vi "test-DiffDriveSim-current.vi"() -> (3 "Test Passed":bool)   [LabVIEW 2019]
uses:
  <vilib>/Rock Robotics/WPI/ThirdParty/JAS_Junk/TrajLib/DCMOTOR.CTL
  <vilib>/Rock Robotics/WPI/ThirdParty/JAS_Junk/TrajLib/LINEAR_SYSTEM.ctl
  <vilib>/Analysis/Matrix/Datatypes/RealMatrix.ctl
  <vilib>/Rock Robotics/WPI/ThirdParty/JAS_Junk/TrajLib/DIFF_DRIVE_TRAIN_SIM.ctl
  <vilib>/Rock Robotics/WPI/ThirdParty/JAS_Junk/TrajLib/DIFF_DRIVE_ToughBoxMini_MotorChoice_ENUM.ctl
  <vilib>/Rock Robotics/WPI/ThirdParty/JAS_Junk/TrajLib/MatBuilder_Create.vi
  <vilib>/Rock Robotics/WPI/ThirdParty/JAS_Junk/TrajLib/LinearSystem_New.vi
  <vilib>/Rock Robotics/WPI/ThirdParty/JAS_Junk/TrajLib/MatBuilder_Fill.vi
  <vilib>/Rock Robotics/WPI/ThirdParty/JAS_Junk/TrajLib/MatrixHelper_Zero.vi
  <vilib>/Rock Robotics/WPI/ThirdParty/JAS_Junk/TrajLib/MatrixHelper_CoerceSize.vi
  <vilib>/Rock Robotics/WPI/ThirdParty/JAS_Junk/TrajLib/Trajectory_Library.lvlib
  <vilib>/Analysis/Matrix/NI_Matrix.lvlib
panel:
  in  "Tab Control":T1(tab)
  out "Left Motor Vel (PV)":dbl format="%20.3f"
  out "Right Motor Vel (PV)":dbl format="%20.3f"
  out "CO Chart":cluster{"Voltage":dbl}(graph)
  out "PV Chart":T2(graph)
  out "Motor Amps":dbl format="%20.3f"
  out "Sim Upd Err":bool
  out "Lin Sys Size Cooerced":bool
  out "Cur Passed 0":bool
  out "Cur Passed 1":bool
  out "Cur Passed 2":bool
  out "DiffDriveMotor":T3 {"Jr_KgM2" format="%13.5p"; "L_H" format="%13.5p"; "Kt_NMPerAmp" format="%13.5p"; "KvINV_RadPerSecPerVolt" format="%13.5p"; "R_Ohms" format="%13.5p"; "FreeSpeed_RadPerSec" format="%13.5p"; "FreeCurrent_Amps" format="%13.5p"; "StallCurrent_Amps" format="%13.5p"; "StallTorque_NM" format="%13.5p"; "nominalVoltage_Volts" format="%13.5p"}
  out "m_DiffDriveVel":T4
  out "Differential Drive Train Sim":T6 {"m_Motor"."Jr_KgM2" format="%13.5p"; "m_Motor"."L_H" format="%13.5p"; "m_Motor"."Kt_NMPerAmp" format="%13.5p"; "m_Motor"."KvINV_RadPerSecPerVolt" format="%13.5p"; "m_Motor"."R_Ohms" format="%13.5p"; "m_Motor"."FreeSpeed_RadPerSec" format="%13.5p"; "m_Motor"."FreeCurrent_Amps" format="%13.5p"; "m_Motor"."StallCurrent_Amps" format="%13.5p"; "m_Motor"."StallTorque_NM" format="%13.5p"; "m_Motor"."nominalVoltage_Volts" format="%13.5p"}
  # "<States,States>"
  # "<States,Inputs>"
  # "<Outputs,States>"
  # "<Outputs,Inputs>"
  # "<States, 1>"
  # "<Outputs, 1>"
  # "<Inputs, 1>"
  # "<Outputs, 1>"
  # "<States,States>"
  # "<States,Inputs>"
  # "<Outputs,States>"
  # "<Outputs,Inputs>"
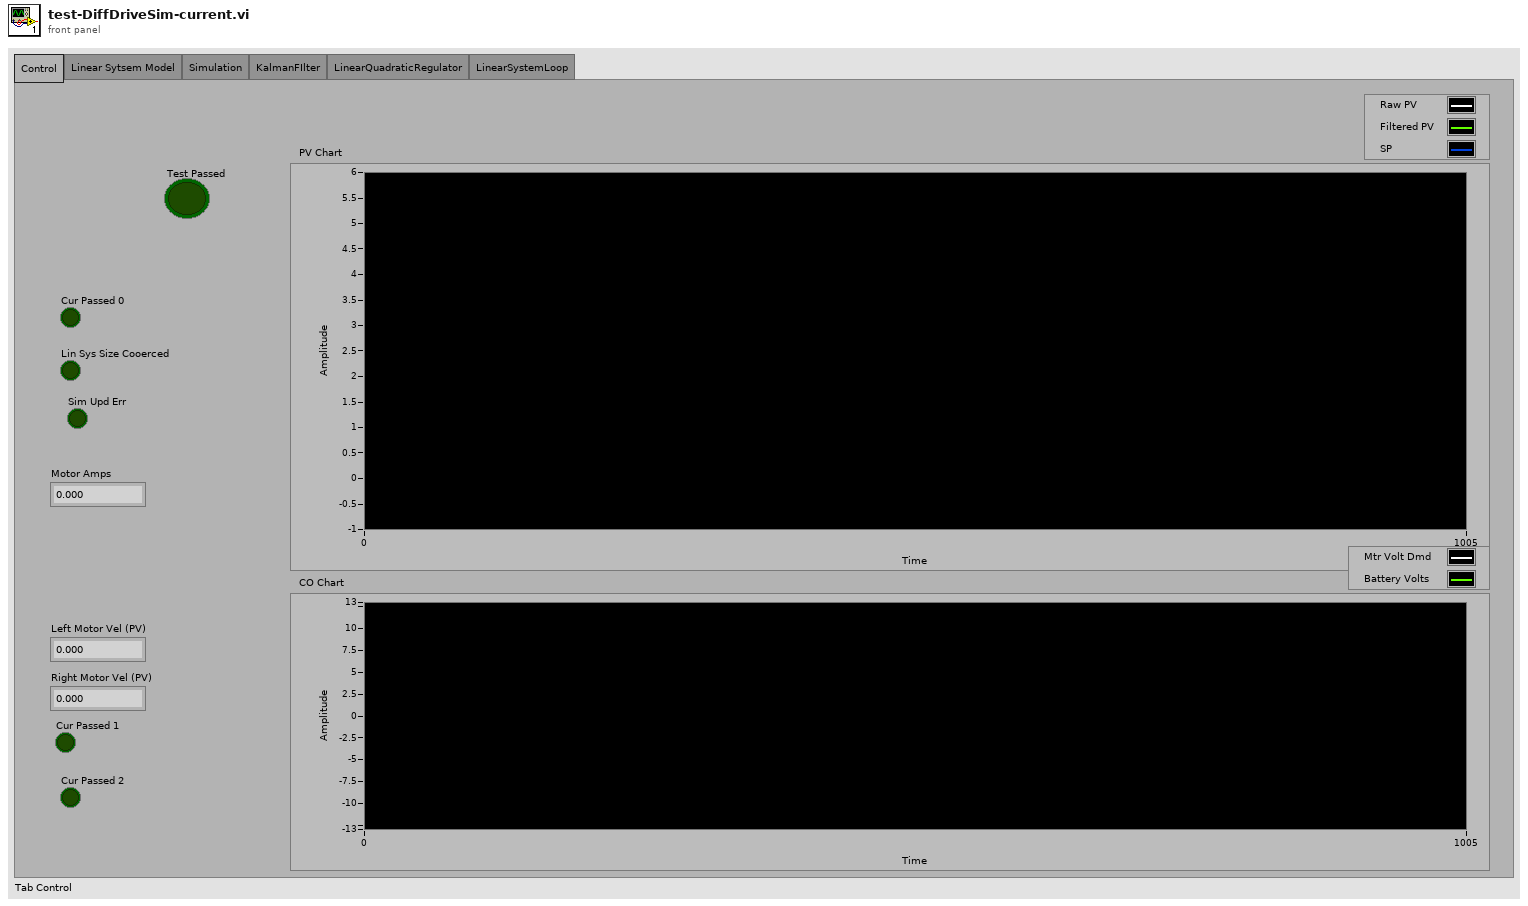
[diagram p1: front panel]
types:
  T1 = enum32{"Control", "Linear Sytsem Model", "Simulation", "KalmanFIlter", "LinearQuadraticRegulator", "LinearSystemLoop"}
  T2 = cluster{"LeftVelocity_M_Per_Sec":dbl, "RightVel_M_Per_Sec":dbl}
  T3 = typedef "Trajectory_Library.lvlib/DCMOTOR.CTL" = cluster{"nominalVoltage_Volts":dbl, "StallTorque_NM":dbl, "StallCurrent_Amps":dbl, "FreeCurrent_Amps":dbl, "FreeSpeed_RadPerSec":dbl, "R_Ohms":dbl, "KvINV_RadPerSecPerVolt":dbl, "Kt_NMPerAmp":dbl, "L_H":dbl, "Jr_KgM2":dbl}
  T4 = typedef "Trajectory_Library.lvlib/LINEAR_SYSTEM.ctl" = cluster{"m_A":T5, "m_B":T5, "m_C":T5, "m_D":T5, "States":i32, "Inputs":i32, "Outputs":i32}
  T5 = typedef "NI_Matrix.lvlib/RealMatrix.ctl" = dbl[][]
  T6 = typedef "Trajectory_Library.lvlib/DIFF_DRIVE_TRAIN_SIM.ctl" = cluster{"m_Plant":T4, "m_X":T5, "m_Y":T5, "m_U":T5, "MeasureStdDev":T5, "m_Motor":T3, "m_OriginalGearing":dbl, "m_CurrentGearing":dbl, "m_WheelRadius_M":dbl, "m_RB":dbl}
  T7 = typedef "Trajectory_Library.lvlib/DIFF_DRIVE_ToughBoxMini_MotorChoice_ENUM.ctl" = enum16{"One CIM Per Side", "Two CIM Per Side", "One MiniCIM Per Side", "Two Mini CIM Per Side", "Two Falcon Per Side", "Two NEO Per Side"}
  T8 = typedef "Trajectory_Library.lvlib/POSE2D.ctl" = cluster{"TRANSLATION":T9, "ROTATION":T10}
  T9 = typedef "Trajectory_Library.lvlib/TRANSLATION2D.ctl" = cluster{"X":dbl, "Y":dbl}
  T10 = typedef "Trajectory_Library.lvlib/ROTATION2D.ctl" = cluster{"VALUE":dbl, "COS":dbl, "SIN":dbl}
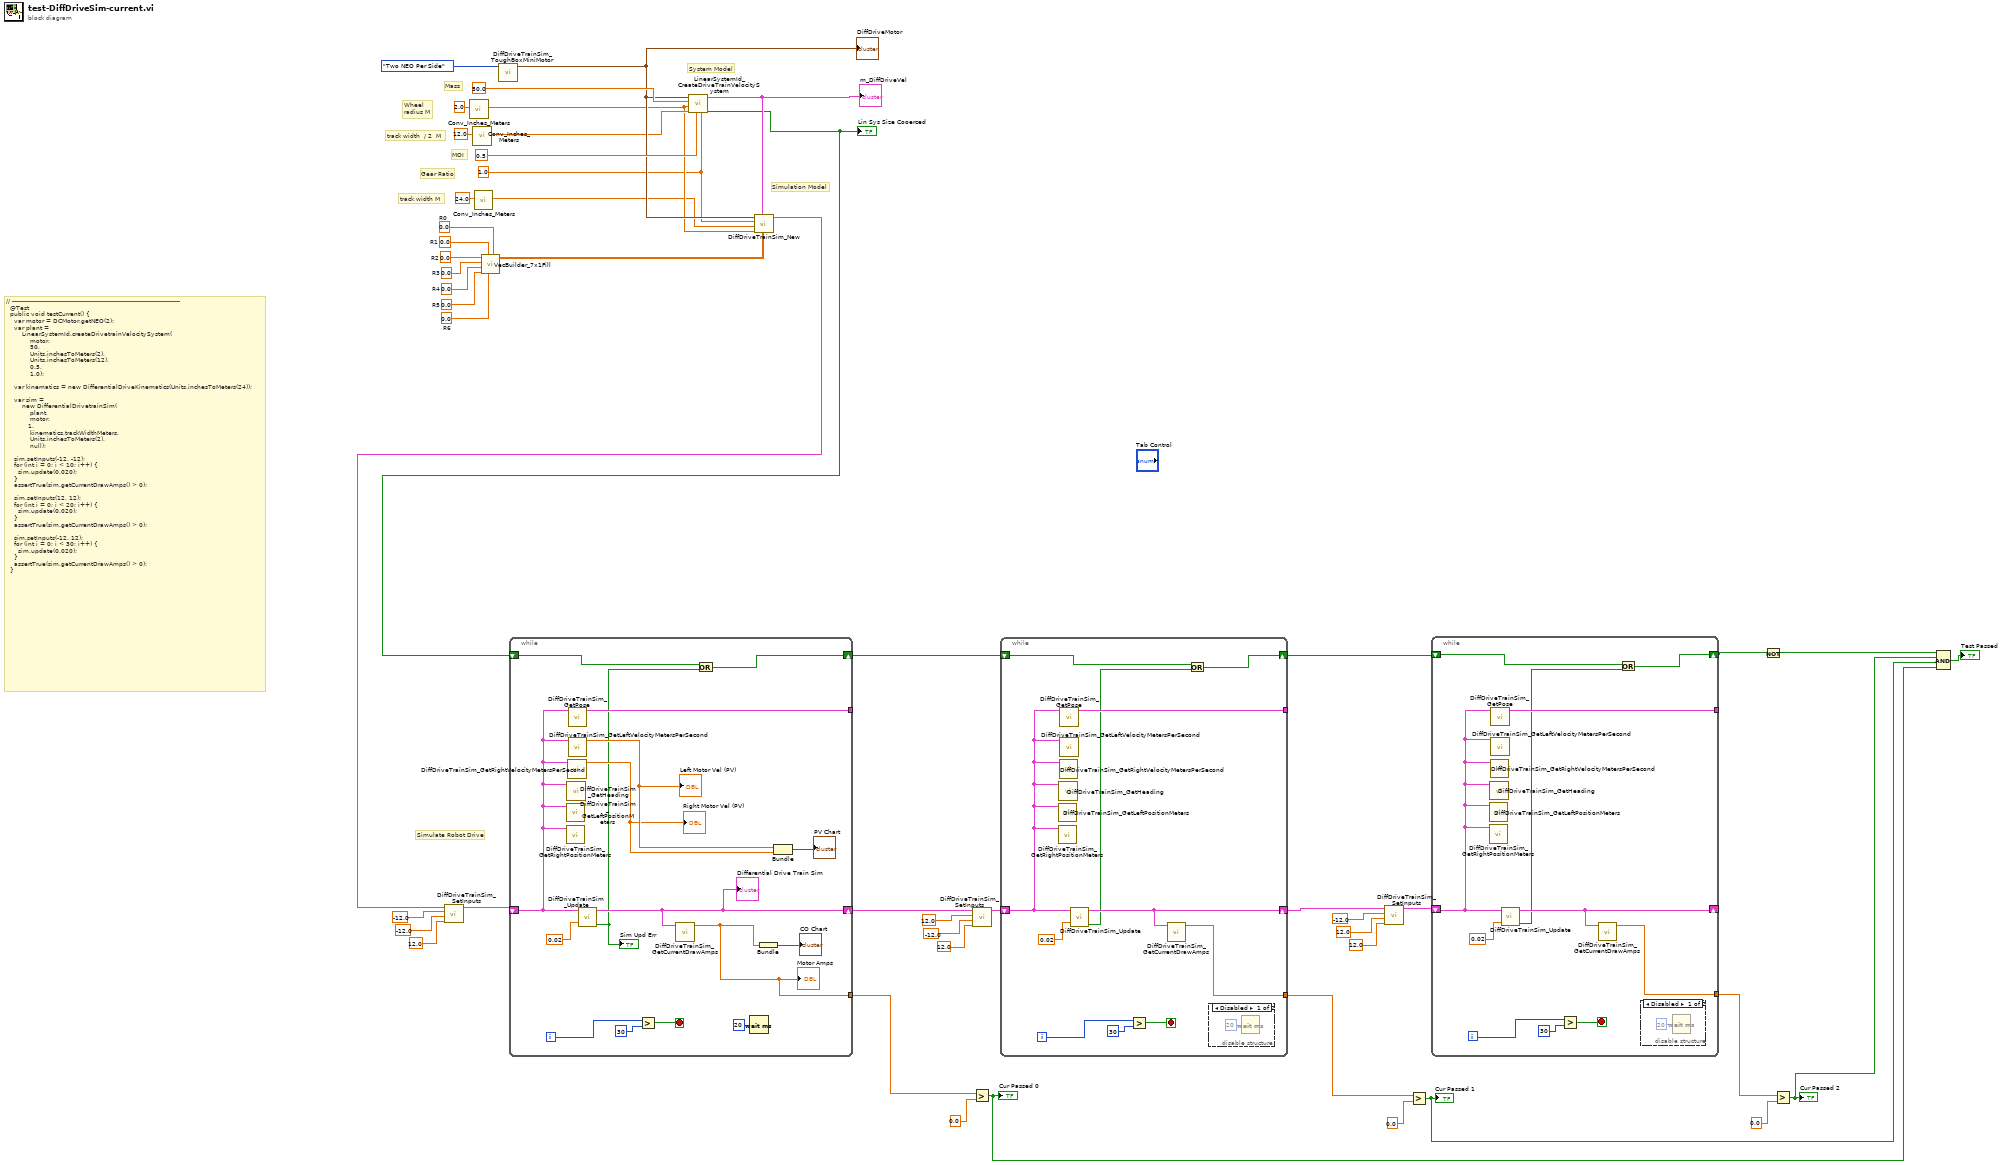
[diagram p0: block diagram]
diagram:
  w38 = 0.0  # R6
  w37 = 0.0  # R5
  w36 = 0.0  # R4
  w35 = 0.0  # R3
  w34 = 0.0  # R2
  w33 = 0.0  # R1
  w32 = 0.0  # R0
  w41 = 1.0 ("G")
  # "// ------------------------------------------------------------------------------------\n  @Test\n  public void testCurrent() {\n    var motor = DCMotor.getNEO(2);\n    var plant =\n        LinearSystemId.createDrivetrainVelocitySystem(\n            motor, \n            50, \n            Units.inchesToMeters(2), \n            Units.inchesToMeters(12), \n            0.5, \n            1.0);\n\n    var kinematics = new DifferentialDriveKinematics(Units.inchesToMeters(24));\n\n    var sim =\n        new DifferentialDrivetrainSim(\n            plant, \n            motor, \n           1, \n            kinematics.trackWidthMeters, \n            Units.inchesToMeters(2), \n            null);\n\n    sim.setInputs(-12, -12);\n    for (int i = 0; i < 10; i++) {\n      sim.update(0.020);\n    }\n    assertTrue(sim.getCurrentDrawAmps() > 0);\n\n    sim.setInputs(12, 12);\n    for (int i = 0; i < 20; i++) {\n      sim.update(0.020);\n    }\n    assertTrue(sim.getCurrentDrawAmps() > 0);\n\n    sim.setInputs(-12, 12);\n    for (int i = 0; i < 30; i++) {\n      sim.update(0.020);\n    }\n    assertTrue(sim.getCurrentDrawAmps() > 0);\n  }"
  # "track width M"
  # "Gear Ratio"
  # "Wheel\nradius M"
  # "track width  / 2  M"
  # "MOI"
  # "Simulation Model"
  # "System Model"
  # "Mass"
  # "Simulate Robot Drive"
  n1 = call <vilib>:"Conv_Inches_Meters.vi"("INCH"=2.0) -> ("Meters"=w43:dbl)  [unwired: 10 in]
  n2 = call <vilib>:"Conv_Inches_Meters.vi"("INCH"=12.0) -> ("Meters"=w44:dbl)  [unwired: 10 in]
  n3 = call <vilib>:"Conv_Inches_Meters.vi"("INCH"=24.0) -> ("Meters"=w39:dbl)  [unwired: 10 in]
  n4 = call <vilib>:"VecBuilder_7x1Fill.vi"("R0"=w32, "R6"=w38, "R1"=w33, "R5"=w37, "R4"=w36, "R3"=w35, "R2"=w34) -> ("output matrix"=w31:T5)  [unwired: 4 in]
  n5 = call <vilib>:"DiffDriveTrainSim_ToughBoxMiniMotor.vi"("ToughBoxMiniMotor"=DIFF_DRIVE_ToughBoxMini_MotorChoice_ENUM."Two NEO Per Side") -> ("DriveMotor"=w45:T3)  [unwired: 10 in]
  "DiffDriveMotor" <- w45
  n6 = call <vilib>:"LinearSystemId_CreateDriveTrainVelocitySystem.vi"("G"=w41, "JKgMetersSquared"=0.5 ("Mass_Kg"), "rbMeters"=w44, "rMeters"=w43, "MassKg"=50.0 ("Mass_Kg"), "Motor"=w45) -> ("Size Coerced"=w24:bool, "Linearsystem"=w42:T4)  [unwired: 4 in]
  "m_DiffDriveVel" <- w42
  "Lin Sys Size Cooerced" <- w24
  n7 = call <vilib>:"DiffDriveTrainSim_New.vi"("MeasurementStdDev"=w31, "DriveTrainPlant"=w42, "WheelRadius_M"=w43, "TrackWidth_M"=w39, "Gearing"=w41, "DriveMotor"=w45) -> ("DiffDriveTrainSim"=w30:T6)  [unwired: 5 in]
  n8 = call <vilib>:"DiffDriveTrainSim_SetInputs.vi"("BatteryVoltage"=12.0, "Right_Volts"=-12.0, "Left_Volts"=-12.0, "in DiffDriveTrainSim"=w30) -> ("out DiffDriveTrainSim"=w29:T6)  [unwired: 6 in, 1 out]
  n9 = while {
    shift-right: [w64] -> w14
    shift-left: w29 -> [w62]
    tunnel: [w55] -> _
    shift-right: [w52] -> w6
    shift-left: w24 -> [w53]
    tunnel: [w51] -> w21
    i -> [w60]
    stop <- w58 stop-if-true
    n10 = call <vilib>:"DiffDriveTrainSim_GetLeftPositionMeters.vi"("DiffDriveTrainSim"=w62) -> ()  [unwired: 10 in, 1 out]
    n11 = call <vilib>:"DiffDriveTrainSim_GetRightPositionMeters.vi"("DiffDriveTrainSim"=w62) -> ()  [unwired: 10 in, 1 out]
    n12 = call <vilib>:"DiffDriveTrainSim_GetHeading.vi"("DiffDriveTrainSim"=w62) -> ()  [unwired: 10 in, 1 out]
    n13 = call <vilib>:"DiffDriveTrainSim_GetRightVelocityMetersPerSecond.vi"("DiffDriveTrainSim"=w62) -> ("RightVel_M_Per_Sec"=w57:dbl)  [unwired: 10 in]
    "Right Motor Vel (PV)" <- w57
    n14 = call <vilib>:"DiffDriveTrainSim_GetPose.vi"("DiffDriveTrainSim"=w62) -> ("Pose"=w55:T8)  [unwired: 10 in]
    n15 = call <vilib>:"DiffDriveTrainSim_GetLeftVelocityMetersPerSecond.vi"("DiffDriveTrainSim"=w62) -> ("LeftVelocity_M_Per_Sec"=w63:dbl)  [unwired: 10 in]
    "Left Motor Vel (PV)" <- w63
    n16 = call <vilib>:"DiffDriveTrainSim_Update.vi"("dT_Seconds"=0.02, "in DiffDriveTrainSim"=w62) -> ("Error"=w54:bool, "out DiffDriveTrainSim"=w64:T6)  [unwired: 8 in]
    "Sim Upd Err" <- w54
    "Differential Drive Train Sim" <- w64
    n17 = Greater?(x=w60, y=30) -> (0:w58:bool)
    n18 = call <vilib>:"DiffDriveTrainSim_GetCurrentDrawAmps.vi"("DiffDriveTrainSim"=w64) -> ("TotalCurrent_Amps"=w51:dbl)  [unwired: 10 in]
    "Motor Amps" <- w51
    n19 = Or(x=w53, y=w54) -> (x .or. y?=w52:bool)
    n20 = Wait (ms)(milliseconds to wait=u32 20) -> ()  [unwired: 1 out]
    n21 = Bundle("TotalCurrent_Amps"=w51) -> (→"CO Chart":cluster{"TotalCurrent_Amps":dbl})  [unwired: 1 in]
    n22 = Bundle("LeftVelocity_M_Per_Sec"=w63, "RightVel_M_Per_Sec"=w57) -> (→"PV Chart":T2)  [unwired: 1 in]
  }
  n23 = call <vilib>:"DiffDriveTrainSim_SetInputs.vi"("BatteryVoltage"=12.0, "Right_Volts"=-12.0, "Left_Volts"=12.0, "in DiffDriveTrainSim"=w14) -> ("out DiffDriveTrainSim"=w13:T6)  [unwired: 6 in, 1 out]
  n24 = Greater?(x=w21, y=0.0) -> (0:w1:bool)
  "Cur Passed 0" <- w1
  n25 = while {
    shift-right: [w76] -> w12
    shift-left: w13 -> [w75]
    tunnel: [w71] -> _
    shift-right: [w68] -> w5
    shift-left: w6 -> [w69]
    tunnel: [w67] -> w8
    i -> [w74]
    stop <- w72 stop-if-true
    n26 = call <vilib>:"DiffDriveTrainSim_GetLeftPositionMeters.vi"("DiffDriveTrainSim"=w75) -> ()  [unwired: 10 in, 1 out]
    n27 = call <vilib>:"DiffDriveTrainSim_GetRightPositionMeters.vi"("DiffDriveTrainSim"=w75) -> ()  [unwired: 10 in, 1 out]
    n28 = call <vilib>:"DiffDriveTrainSim_GetHeading.vi"("DiffDriveTrainSim"=w75) -> ()  [unwired: 10 in, 1 out]
    n29 = call <vilib>:"DiffDriveTrainSim_GetRightVelocityMetersPerSecond.vi"("DiffDriveTrainSim"=w75) -> ()  [unwired: 10 in, 1 out]
    n30 = call <vilib>:"DiffDriveTrainSim_GetPose.vi"("DiffDriveTrainSim"=w75) -> ("Pose"=w71:T8)  [unwired: 10 in]
    n31 = call <vilib>:"DiffDriveTrainSim_GetLeftVelocityMetersPerSecond.vi"("DiffDriveTrainSim"=w75) -> ()  [unwired: 10 in, 1 out]
    n32 = call <vilib>:"DiffDriveTrainSim_Update.vi"("dT_Seconds"=0.02, "in DiffDriveTrainSim"=w75) -> ("Error"=w70:bool, "out DiffDriveTrainSim"=w76:T6)  [unwired: 8 in]
    n33 = Greater?(x=w74, y=30) -> (0:w72:bool)
    n34 = call <vilib>:"DiffDriveTrainSim_GetCurrentDrawAmps.vi"("DiffDriveTrainSim"=w76) -> ("TotalCurrent_Amps"=w67:dbl)  [unwired: 10 in]
    n35 = Or(x=w69, y=w70) -> (x .or. y?=w68:bool)
    n36 = disable-structure shown="Disabled" {
      frame Disabled {
        n37 = Wait (ms)(milliseconds to wait=u32 20) -> ()  [unwired: 1 out]
      }
      frame Enabled {
      }
    }
  }
  n38 = call <vilib>:"DiffDriveTrainSim_SetInputs.vi"("BatteryVoltage"=12.0, "Right_Volts"=12.0, "Left_Volts"=-12.0, "in DiffDriveTrainSim"=w12) -> ("out DiffDriveTrainSim"=w11:T6)  [unwired: 6 in, 1 out]
  n39 = Greater?(x=w8, y=0.0) -> (0:w2:bool)
  "Cur Passed 1" <- w2
  n40 = while {
    shift-right: [w88] -> _
    shift-left: w11 -> [w87]
    tunnel: [w83] -> _
    shift-right: [w80] -> w4
    shift-left: w5 -> [w81]
    tunnel: [w79] -> w7
    i -> [w86]
    stop <- w84 stop-if-true
    n41 = call <vilib>:"DiffDriveTrainSim_GetLeftPositionMeters.vi"("DiffDriveTrainSim"=w87) -> ()  [unwired: 10 in, 1 out]
    n42 = call <vilib>:"DiffDriveTrainSim_GetRightPositionMeters.vi"("DiffDriveTrainSim"=w87) -> ()  [unwired: 10 in, 1 out]
    n43 = call <vilib>:"DiffDriveTrainSim_GetHeading.vi"("DiffDriveTrainSim"=w87) -> ()  [unwired: 10 in, 1 out]
    n44 = call <vilib>:"DiffDriveTrainSim_GetRightVelocityMetersPerSecond.vi"("DiffDriveTrainSim"=w87) -> ()  [unwired: 10 in, 1 out]
    n45 = call <vilib>:"DiffDriveTrainSim_GetPose.vi"("DiffDriveTrainSim"=w87) -> ("Pose"=w83:T8)  [unwired: 10 in]
    n46 = call <vilib>:"DiffDriveTrainSim_GetLeftVelocityMetersPerSecond.vi"("DiffDriveTrainSim"=w87) -> ()  [unwired: 10 in, 1 out]
    n47 = call <vilib>:"DiffDriveTrainSim_Update.vi"("dT_Seconds"=0.02, "in DiffDriveTrainSim"=w87) -> ("Error"=w82:bool, "out DiffDriveTrainSim"=w88:T6)  [unwired: 8 in]
    n48 = Greater?(x=w86, y=30) -> (0:w84:bool)
    n49 = call <vilib>:"DiffDriveTrainSim_GetCurrentDrawAmps.vi"("DiffDriveTrainSim"=w88) -> ("TotalCurrent_Amps"=w79:dbl)  [unwired: 10 in]
    n50 = Or(x=w81, y=w82) -> (x .or. y?=w80:bool)
    n51 = disable-structure shown="Disabled" {
      frame Disabled {
        n52 = Wait (ms)(milliseconds to wait=u32 20) -> ()  [unwired: 1 out]
      }
      frame Enabled {
      }
    }
  }
  n53 = Not(x=w4) -> (.not. x?=w23:bool)
  n54 = Greater?(x=w7, y=0.0) -> (0:w3:bool)
  "Cur Passed 2" <- w3
  n55 = Compound Arithmetic op=AND(w23, w3, w2, w1) -> (→"Test Passed":bool)
